vi "Read_CAL_PARAMETER_Connector_B.vi"() -> ()   [LabVIEW 2016]
doc: "The myRIO Project template acquires acceleration data from the onboard accelerometer and displays the changes of acceleration values in a waveform chart."
uses:
  <vilib>/myRIO/Common/Instrument Driver Framework/Utilities/typedefs/Generic FPGA Reference.ctl
  <vilib>/myRIO/Common/Instrument Driver Framework/Utilities/typedefs/myRIO v1.0 Reference.ctl
  <vilib>/myRIO/Common/Instrument Driver Framework/Utilities/typedefs/Hardware Version Enum.ctl
  <vilib>/myRIO/Common/Instrument Driver Framework/Utilities/typedefs/myRIO Generic Hardware Reference.ctl
  <vilib>/myRIO/Common/Instrument Driver Framework/Utilities/vis/Is FPGA Ref Available.vi
  <vilib>/userdefined/High Color/nirio_resource_hc.ctl
  <vilib>/myRIO/Express VI/Onboard IO/I2C/I2C Express VI.xnode
  <vilib>/myRIO/Instrument Drivers/Onboard IO/I2C/vis/Configure.vi
  <vilib>/myRIO/Instrument Drivers/Onboard IO/I2C/I2C.lvlib
  <vilib>/myRIO/Instrument Drivers/Onboard IO/I2C/vis/Write Read.vi
  <vilib>/myRIO/Instrument Drivers/Onboard IO/I2C/typedefs/I2C Transfer Rate.ctl
  <vilib>/myRIO/Instrument Drivers/Onboard IO/I2C/typedefs/I2C User Configuration.ctl
  <vilib>/myRIO/Instrument Drivers/Onboard IO/I2C/typedefs/I2C Configuration.ctl
  <vilib>/myRIO/Common/Instrument Driver Framework/myRIO v1.0/I2C/typedefs/I2C Channels Enum.ctl
  <vilib>/myRIO/Instrument Drivers/Onboard IO/I2C/typedefs/I2C Reference.ctl
  <vilib>/myRIO/Instrument Drivers/Onboard IO/I2C/vis/myRIO I2C Open.xnode
  <vilib>/myRIO/Common/Instrument Driver Framework/myRIO v1.0/I2C/vis/myRIO v1.1 Open I2C.vi
  <vilib>/myRIO/Instrument Drivers/Onboard IO/I2C/vis/Write.vi
panel:
  out "16bit integer":i16[](array[numeric])
  out "x*2^n":dbl[](array[numeric])
  out "Array 3":i16[][](array[numeric])
  out "subarray 4":u16[](array[numeric])
  out "subarray 3":u16[](array[numeric])
  out "subarray 2":u16[](array[numeric])
  out "subarray":u16[](array[numeric])
  out "error out":errorcluster
  out "UP_Value":u16[](array[numeric])
  out "Numerisches Bedienelement":i32
  out "Array 2":i16[][](array[numeric])
  out "UT_Value":u16[](array[numeric])
  out "READ LSB CAL_PARAM":u8[][](array[numeric]) format="%.0x"
  out "READ MSB CAL_PARAM":u8[][](array[numeric]) format="%.0x"
  out "Device_ID":u8[](array[numeric]) format="%.0x"
  in  "Stop":bool
  # "Device is connceted to MXI connector B of the myRIO"
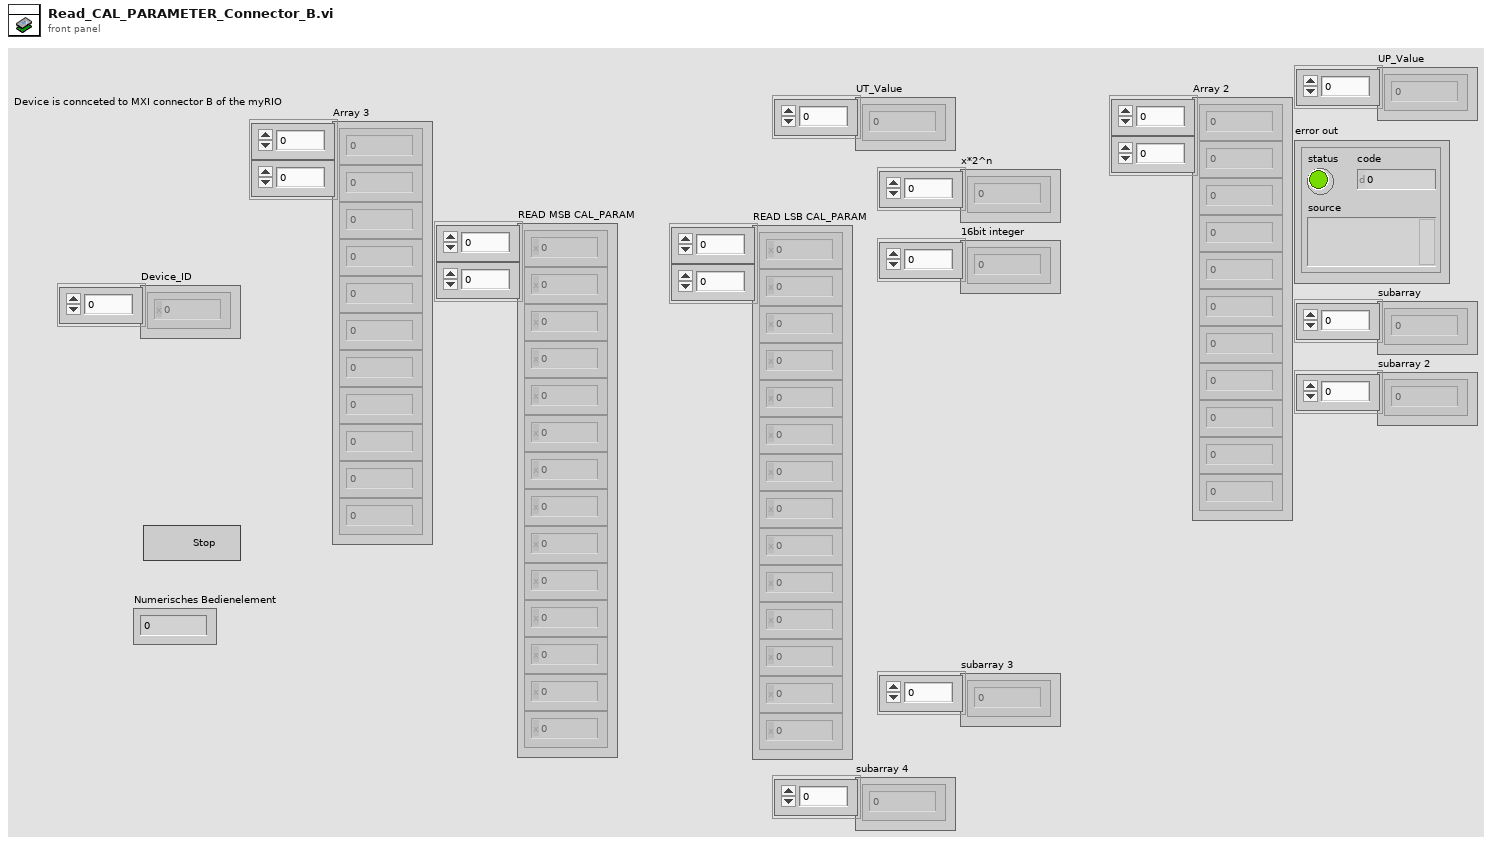
[diagram p1: front panel]
types:
  T1 = typedef "I2C.lvlib/I2C Reference.ctl" = cluster{"myRIO Reference":T2, "I2C Channels Enum":T6, "I2C Configuration":T7}
  T2 = typedef "myRIO Generic Hardware Reference.ctl" = cluster{"myRIO Model":T3, "myRIO Hardware Reference":T4}
  T3 = typedef "Hardware Version Enum.ctl" = enum16{"Unknown", "myRIO-1900", "myRIO-1950", "roboRIO", "NI ELVIS RIO CM"}
  T4 = typedef "myRIO v1.0 Reference.ctl" = cluster{"Generic FPGA Reference":T5, "Allow multiple opens":bool}
  T5 = typedef "Generic FPGA Reference.ctl" = refnum<k20>
  T6 = typedef "I2C Channels Enum.ctl" = enum16{"Not Connected", "A/I2C", "B/I2C", "I2C/I2C"}
  T7 = typedef "I2C.lvlib/I2C Configuration.ctl" = cluster{"I2C Transfer Rate":T8}
  T8 = typedef "I2C.lvlib/I2C Transfer Rate.ctl" = enum16{"Standard mode (100 kbps)", "Fast mode (400 kbps)"}
  T9 = typedef "I2C.lvlib/I2C User Configuration.ctl" = cluster{"I2C Transfer Rate":T8}
  T10 = typedef "nirio_resource_hc.ctl" = tag
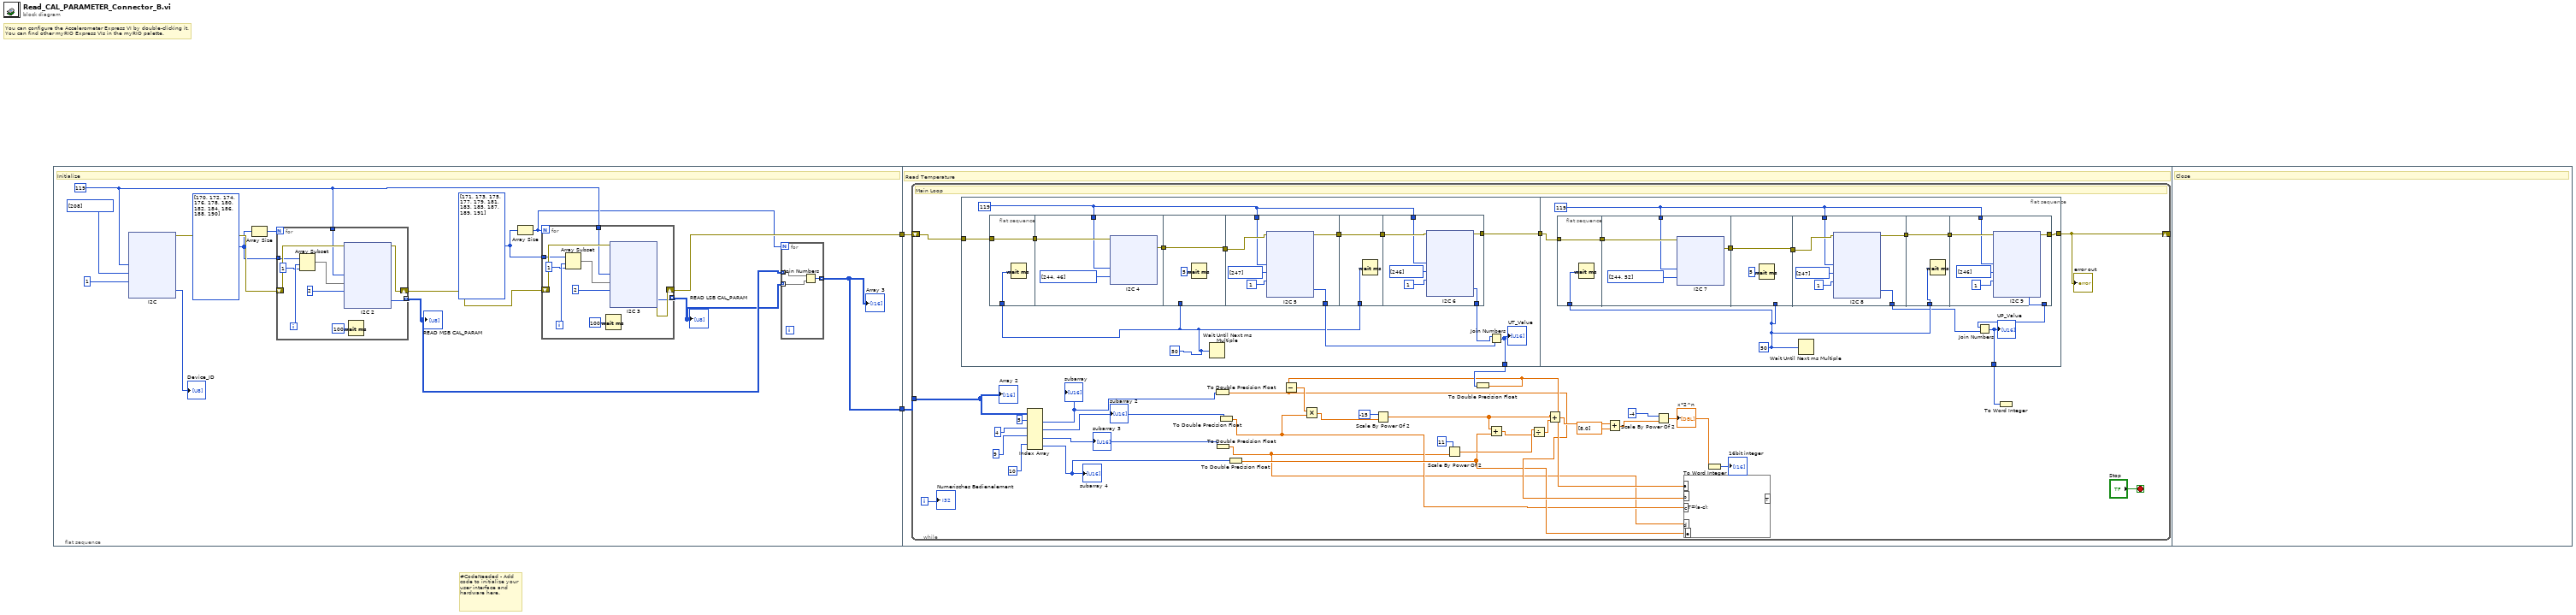
[diagram p0: block diagram]
diagram:
  # "#CodeNeeded - Add code to initialize your user interface and hardware here."
  # "You can configure the Accelerometer Express VI by double-clicking it.\nYou can find other myRIO Express VIs in the myRIO palette."
  n1 = flat-sequence {
    tunnel: [w7] -> w2
    tunnel: [w3] -> w1
    tunnel: w2 -> [w161]
    tunnel: w1 -> [w160]
    frame #0 {
      w10 = u8[] [171, 173, 175, 177, 179, 181, 183, 185, 187, 189, 191] ("Slave Address (7-bit)")
      w11 = u8[] [170, 172, 174, 176, 178, 180, 182, 184, 186, 188, 190] ("Slave Address (7-bit)")
      w9 = u8 119 ("Slave Address (7-bit)")
      # "Initialize"
      n2 = xnode "I2C"("Slave Address (7-bit)"=w9, "Bytes to Write"=u8[] [208] ("Slave Address (7-bit)"), "Byte Count"=u32 1) -> ("Bytes Read"=→"Device_ID":u8[], "error out"=w13:errorcluster)  [unwired: 1 in]
      n3 = Array Size(array=w11) -> (size(s)=w12:i32)
      n4 = for {
        N: w12 -> [_]
        tunnel: w9 -> [w77]
        shift-right: [w78] -> w8
        shift-left: w13 -> [w79]
        tunnel: [w76] -> w5 mode=indexing
        tunnel: w11 -> [w74]
        i -> [w72]
        n5 = Array Subset(array=w74, index=w72, length=1 ("Länge")) -> (w73:u8[])
        n6 = xnode "I2C 2"("Slave Address (7-bit)"=w77, "Bytes to Write"=w73, "Byte Count"=u32 2, "error in (no error)"=w79) -> ("Bytes Read"=w76:u8[], "error out"=w78:errorcluster)
        n7 = Wait (ms)(milliseconds to wait=u32 100 ("Zu wartende ms")) -> ()  [unwired: 1 out]
      }
      "READ MSB CAL_PARAM" <- w5
      n8 = Array Size(array=w10) -> (size(s)=w6:i32)
      n9 = for {
        N: w6 -> [_]
        tunnel: w9 -> [w27]
        shift-right: [w28] -> w7
        shift-left: w8 -> [w29]
        tunnel: [w26] -> w4 mode=indexing
        tunnel: w10 -> [w24]
        i -> [w22]
        n10 = Array Subset(array=w24, index=w22, length=1 ("Länge")) -> (w23:u8[])
        n11 = Wait (ms)(milliseconds to wait=u32 100 ("Zu wartende ms")) -> ()  [unwired: 1 out]
        n12 = xnode "I2C 3"("Slave Address (7-bit)"=w27, "Bytes to Write"=w23, "Byte Count"=u32 2, "error in (no error)"=w29) -> ("Bytes Read"=w26:u8[], "error out"=w28:errorcluster)
      }
      "READ LSB CAL_PARAM" <- w4
      n13 = for {
        N: w6 -> [_]
        tunnel: w5 -> [w19] mode=indexing
        tunnel: w4 -> [w18] mode=indexing
        tunnel: [w17] -> w3 mode=indexing
        n14 = Join Numbers(hi=w19, lo=w18) -> ((hi.lo)=w17:u16[])
      }
      "Array 3" <- w3
    }
    frame #1 {
      # "Read Temperature"
      n15 = while {
        shift-right: [w192] -> _
        shift-left: w161 -> [w195]
        tunnel: w160 -> [w190]
        i -> [w194]
        stop <- "Stop" stop-if-true
        # "Main Loop"
        n16 = flat-sequence {
          tunnel: w195 -> [w203]
          tunnel: [w201] -> w193
          tunnel: [w197] -> w173
          tunnel: [w354] -> w192
          tunnel: w193 -> [w355]
          tunnel: [w349] -> w191
          frame #0 {
            w198 = u32 50 ("milliseconds to wait")
            w202 = u8 119 ("Slave Address (7-bit)")
            n17 = flat-sequence {
              tunnel: w203 -> [w210]
              tunnel: [w210] -> w208
              tunnel: w198 -> [w209]
              tunnel: [w213] -> w207
              tunnel: w202 -> [w211]
              tunnel: w208 -> [w212]
              tunnel: [w254] -> w206
              tunnel: w207 -> [w254]
              tunnel: w198 -> [_]
              tunnel: w206 -> [w258]
              tunnel: [w257] -> w199
              tunnel: [w256] -> w205
              tunnel: w202 -> [w255]
              tunnel: w205 -> [w302]
              tunnel: [w302] -> w204
              tunnel: w198 -> [w301]
              tunnel: w204 -> [w306]
              tunnel: [w305] -> w201
              tunnel: [w304] -> w200
              tunnel: w202 -> [w303]
              frame #0 {
                n18 = Wait (ms)(milliseconds to wait=w209) -> ()  [unwired: 1 out]
              }
              frame #1 {
                n19 = xnode "I2C 4"("Slave Address (7-bit)"=w211, "Bytes to Write"=u8[] [244, 46], "error in (no error)"=w212) -> ("error out"=w213:errorcluster)
              }
              frame #2 {
                n20 = Wait (ms)(milliseconds to wait=u32 5 ("Zu wartende ms")) -> ()  [unwired: 1 out]
              }
              frame #3 {
                n21 = xnode "I2C 5"("Slave Address (7-bit)"=w255, "Bytes to Write"=u8[] [247], "Byte Count"=u8 1 ("Slave Address (7-bit)"), "error in (no error)"=w258) -> ("Bytes Read"=w257:u8[], "error out"=w256:errorcluster)
              }
              frame #4 {
                n22 = Wait (ms)(milliseconds to wait=w301) -> ()  [unwired: 1 out]
              }
              frame #5 {
                n23 = xnode "I2C 6"("Slave Address (7-bit)"=w303, "Bytes to Write"=u8[] [246], "Byte Count"=u8 1 ("Slave Address (7-bit)"), "error in (no error)"=w306) -> ("Bytes Read"=w304:u8[], "error out"=w305:errorcluster)
              }
            }
            n24 = Wait Until Next ms Multiple(millisecond multiple=w198) -> ()  [unwired: 1 out]
            n25 = Join Numbers(hi=w200, lo=w199) -> ((hi.lo)=w197:u16[])
            "UT_Value" <- w197
          }
          frame #1 {
            w352 = u32 50 ("milliseconds to wait")
            w353 = u8 119 ("Slave Address (7-bit)")
            n26 = flat-sequence {
              tunnel: w355 -> [w362]
              tunnel: [w362] -> w360
              tunnel: w352 -> [w361]
              tunnel: [w365] -> w359
              tunnel: w353 -> [w363]
              tunnel: w360 -> [w364]
              tunnel: [w406] -> w358
              tunnel: w359 -> [w406]
              tunnel: w352 -> [_]
              tunnel: w358 -> [w410]
              tunnel: [w409] -> w351
              tunnel: [w408] -> w357
              tunnel: w353 -> [w407]
              tunnel: w357 -> [w454]
              tunnel: [w454] -> w356
              tunnel: w352 -> [w453]
              tunnel: w356 -> [w458]
              tunnel: [w457] -> w354
              tunnel: [w455] -> _
              tunnel: w353 -> [w456]
              tunnel: [w455] -> w350
              frame #0 {
                n27 = Wait (ms)(milliseconds to wait=w361) -> ()  [unwired: 1 out]
              }
              frame #1 {
                n28 = xnode "I2C 7"("Slave Address (7-bit)"=w363, "Bytes to Write"=u8[] [244, 52], "error in (no error)"=w364) -> ("error out"=w365:errorcluster)
              }
              frame #2 {
                n29 = Wait (ms)(milliseconds to wait=u32 5 ("Zu wartende ms")) -> ()  [unwired: 1 out]
              }
              frame #3 {
                n30 = xnode "I2C 8"("Slave Address (7-bit)"=w407, "Bytes to Write"=u8[] [247], "Byte Count"=u8 1 ("Slave Address (7-bit)"), "error in (no error)"=w410) -> ("Bytes Read"=w409:u8[], "error out"=w408:errorcluster)
              }
              frame #4 {
                n31 = Wait (ms)(milliseconds to wait=w453) -> ()  [unwired: 1 out]
              }
              frame #5 {
                n32 = xnode "I2C 9"("Slave Address (7-bit)"=w456, "Bytes to Write"=u8[] [246], "Byte Count"=u8 1 ("Slave Address (7-bit)"), "error in (no error)"=w458) -> ("Bytes Read"=w455:u8[], "error out"=w457:errorcluster)
              }
            }
            n33 = Wait Until Next ms Multiple(millisecond multiple=w352) -> ()  [unwired: 1 out]
            n34 = Join Numbers(hi=w350, lo=w351) -> ((hi.lo)=w349:u16[])
            "UP_Value" <- w349
          }
        }
        n35 = Index Array(array=w190, index (row) #1=5 ("index (row)"), index (row) #2=4, index (row) #3=9, index (row) #4=10) -> (element #1=w185:u16[], element #2=w184:u16[], element #3=w183:u16[], element #4=w182:u16[])  [unwired: 4 in]
        "subarray" <- w185
        "subarray 2" <- w184
        "subarray 3" <- w183
        "subarray 4" <- w182
        n36 = To Double Precision Float(number=w185) -> (double precision float=w165:dbl[])
        n37 = To Double Precision Float(number=w183) -> (double precision float=w162:dbl[])
        n38 = To Double Precision Float(number=w184) -> (double precision float=w163:dbl[])
        n39 = To Double Precision Float(number=w182) -> (double precision float=w164:dbl[])
        n40 = Scale By Power Of 2(n=i16 11, x=w162) -> (x*2^n=w176:dbl[])
        n41 = To Double Precision Float(number=w173) -> (double precision float=w166:dbl[])
        n42 = Subtract(x=w166, y=w165) -> (x-y=w181:dbl[])
        n43 = Multiply(x=w181, y=w163) -> (x*y=w180:dbl[])
        n44 = Scale By Power Of 2(n=i16 -15, x=w180) -> (x*2^n=w177:dbl[])
        n45 = Add(x=w177, y=w164) -> (x+y=w175:dbl[])
        n46 = Divide(x=w176, y=w175) -> (x/y=w172:dbl[])
        n47 = Add(x=w177, y=w172) -> (x+y=w174:dbl[])
        n48 = Add(x=w174, y=dbl[] [8.0]) -> (x+y=w169:dbl[])
        n49 = Scale By Power Of 2(n=i16 -4, x=w169) -> (x*2^n=w168:dbl[])
        "x*2^n" <- w168
        n50 = formula code="T=(a-c);"("b"=w165, "d"=w162, "e"=w164, "a"=w166, "c"=w163) -> ()  [unwired: 1 out]
        n51 = To Word Integer(number=w168) -> (16bit integer=→"16bit integer":i16[])
        n52 = To Word Integer(number=w191) -> ()  [unwired: 1 out]
        "Numerisches Bedienelement" <- w194
        "error out" <- w192
        "Array 2" <- w190
      }
    }
    frame #2 {
      # "Close"
    }
  }
